vi "WSVCAP SHL Host LL RFFE Build and Parse Data.vi"(0 "Data Out":string, 1 "Data Out (Cycle Commands)":string[](array[string]), 2 "Post Command Delay":dbl[](array[numeric]) format="%#.0p s", 7 "Clock Rate (Hz) (Cycle Only)":dbl=50000.0, 9 "RFFE Data In [U8]":u8[][](array[numeric]) format="%02x", 12 "Simulate FPGA (Cycle Only)":bool, 13 "DUT Mask (All)":bool[](array[boolean])=[TRUE, TRUE, TRUE, TRUE, TRUE, TRUE, TRUE, TRUE, TRUE, TRUE, TRUE, TRUE, TRUE, TRUE, TRUE, TRUE, TRUE, TRUE, TRUE, TRUE, TRUE, TRUE, TRUE, TRUE, TRUE, TRUE, TRUE, TRUE, TRUE, TRUE, TRUE, TRUE, TRUE, TRUE, TRUE, TRUE, TRUE, TRUE, TRUE, TRUE, TRUE, TRUE, TRUE, TRUE, TRUE, TRUE, TRUE, TRUE, TRUE, TRUE, TRUE, TRUE, TRUE, TRUE, TRUE, TRUE, TRUE, TRUE, TRUE, TRUE, TRUE, TRUE, TRUE, TRUE]) -> (4 "RFFE Data Out [U8]":u8[][](array[numeric]) format="%02x", 6 "CMD Lengths (Bits)":u8[](array[numeric]), 8 "CMD Delays (Ticks)":u32[](array[numeric]), 10 "RFFE Data In":string[](array[string]))   [LabVIEW 2017]
panel:
  # "DUT 01"
  # "DUT 02"
  # "DUT 03"
  # "DUT 04"
  # "DUT 05"
  # "DUT 06"
  # "DUT 07"
  # "DUT 08"
  # "DUT 09"
  # "DUT 10"
  # "DUT 11"
  # "DUT 12"
  # "DUT 13"
  # "DUT 14"
  # "DUT 15"
  # "DUT 16"
  # "DUT 17"
  # "DUT 18"
  # "DUT 19"
  # "DUT 20"
  # "DUT 21"
  # "DUT 22"
  # "DUT 23"
  # "DUT 24"
  # "DUT 25"
  # "DUT 26"
  # "DUT 27"
  # "DUT 28"
  # "DUT 29"
  # "DUT 30"
  # "DUT 31"
  # "DUT 32"
  # "DUT 33"
  # "DUT 34"
  # "DUT 35"
  # "DUT 36"
  # "DUT 37"
  # "DUT 38"
  # "DUT 39"
  # "DUT 40"
  # "DUT 41"
  # "DUT 42"
  # "DUT 43"
  # "DUT 44"
  # "DUT 45"
  # "DUT 46"
  # "DUT 47"
  # "DUT 48"
  # "DUT 49"
  # "DUT 50"
  # "DUT 51"
  # "DUT 52"
  # "DUT 53"
  # "DUT 54"
  # "DUT 55"
  # "DUT 56"
  # "DUT 57"
  # "DUT 58"
  # "DUT 59"
  # "DUT 60"
  # "DUT 61"
  # "DUT 62"
  # "DUT 63"
  # "DUT 64"
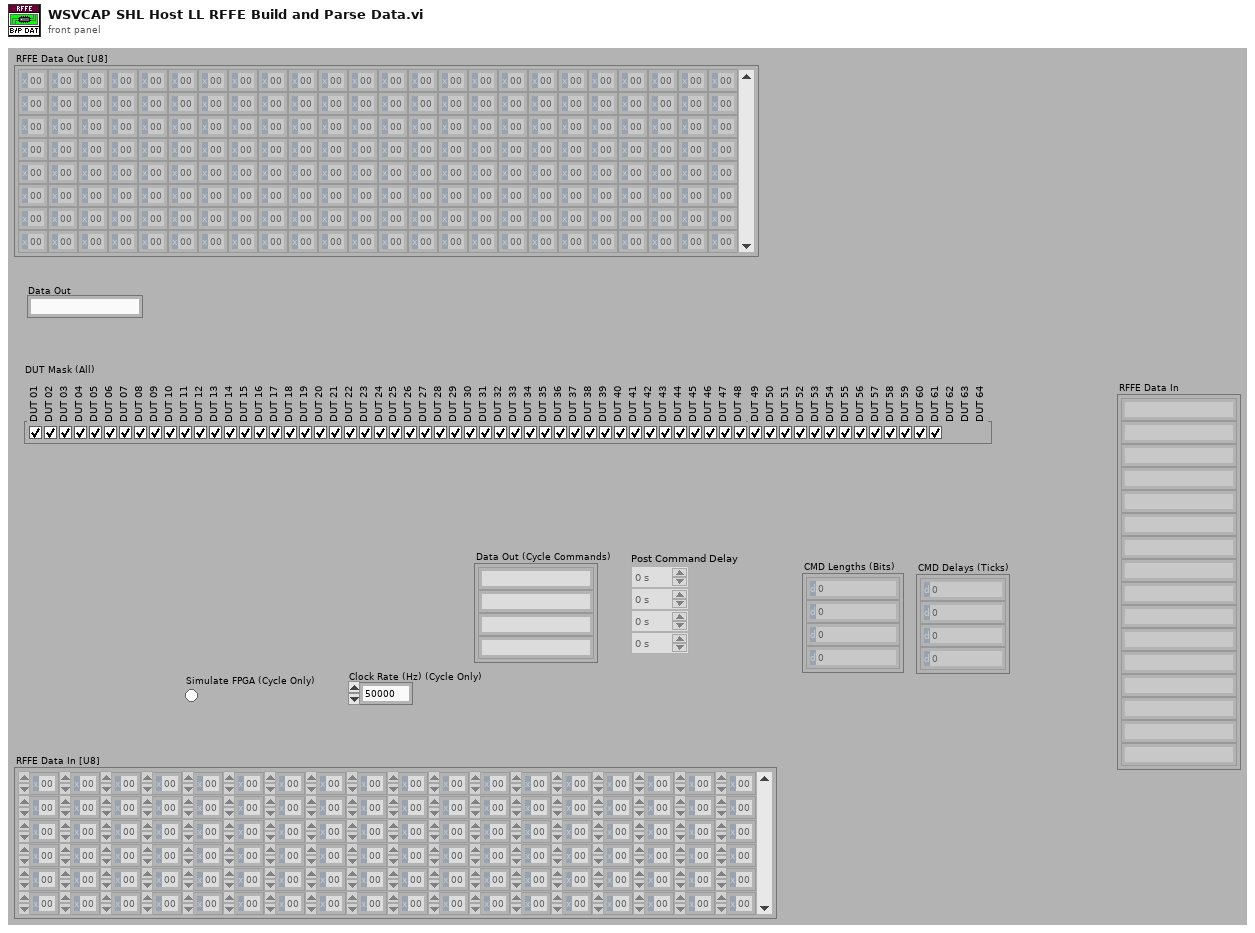
[diagram p1: front panel]
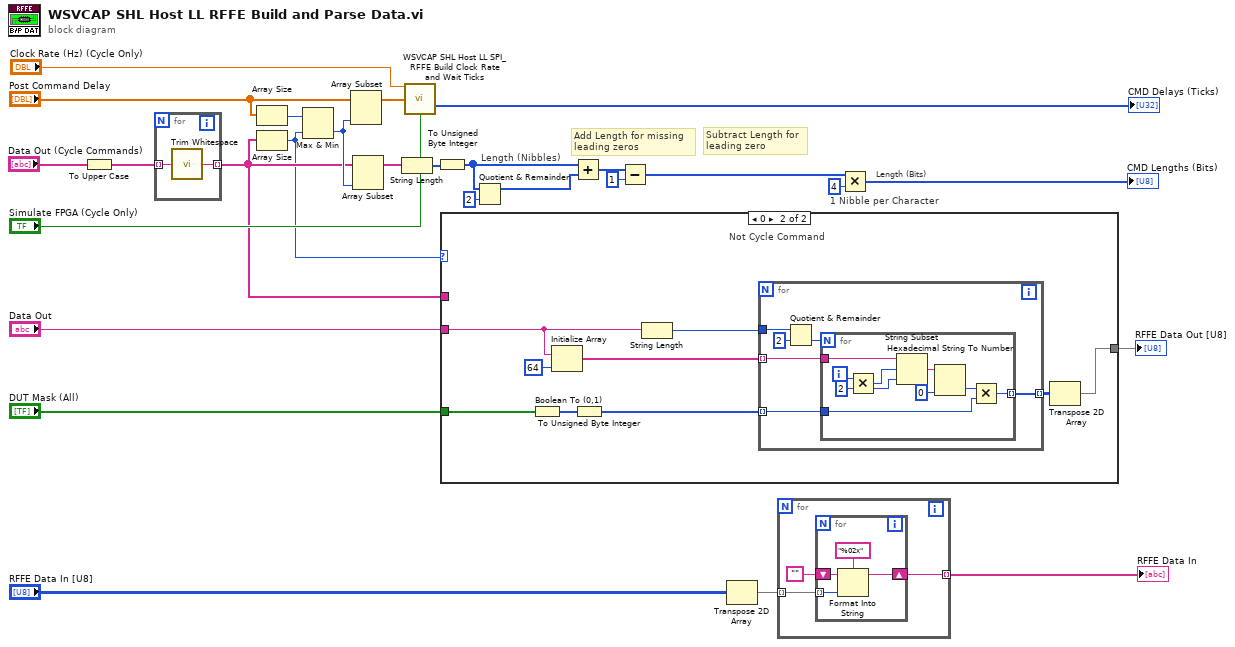
[diagram p0: block diagram]
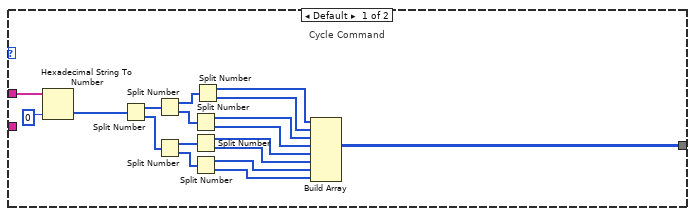
[diagram p2: hidden frame]
diagram:
  # "Subtract Length for\nleading zero"
  # "Add Length for missing\nleading zeros"
  # "Length (Bits)"
  # "Length (Nibbles)"
  # "1 Nibble per Character"
  n1 = To Upper Case(1:"Data Out (Cycle Commands)") -> (0:w2:string[])
  n2 = for {
    tunnel: w2 -> [w29] mode=indexing
    tunnel: [w28] -> w12 mode=indexing
    n3 = call <vilib>:"Trim Whitespace.vi"("string"=w29) -> ("trimmed string"=w28:string)  [unwired: 1 in]
  }
  n4 = Array Size(array="Post Command Delay") -> (size(s)=w21:i32)
  n5 = Array Size(array=w12) -> (size(s)=w11:i32)
  n6 = Max & Min(x=w21, y=w11) -> (min(x,y)=w18:i32)  [unwired: 1 out]
  n7 = Array Subset(array="Post Command Delay", length=w18) -> (w19:dbl[])  [unwired: 1 in]
  n8 = Array Subset(array=w12, length=w18) -> (w17:string[])  [unwired: 1 in]
  n9 = String Length(string=w17) -> (length=w23:i32[])
  n10 = call "WSVCAP SHL Host LL SPI_RFFE Build Clock Rate and Wait Ticks.vi"("Clock Rate (Hz)"="Clock Rate (Hz) (Cycle Only)", "CMD Delay (s)"=w19, "Simulate FPGA"="Simulate FPGA (Cycle Only)") -> ("CMD Delay (Ticks)"=→"CMD Delays (Ticks)":u32[])  [unwired: 9 in, 3 out]
  n11 = To Unsigned Byte Integer(number=w23) -> (unsigned 8bit integer=w8:u8[])
  n12 = case shown="0" w11 {
    tunnel: "DUT Mask (All)" -> [_ w56]
    tunnel: [w30 w51] -> w24
    tunnel: "Data Out" -> [_ w49]
    tunnel: w12 -> [w47 _]
    frame Default {
      # "Cycle Command"
      n13 = Hexadecimal String To Number(string=w47, default (0uL)=u64 0 ("Read Data")) -> (number=w40:u64[])  [unwired: 1 in, 1 out]
      n14 = Split Number(x=w40) -> (hi(x)=w45:u32[], lo(x)=w44:u32[])
      n15 = Split Number(x=w45) -> (hi(x)=w33:u16[], lo(x)=w43:u16[])
      n16 = Split Number(x=w44) -> (hi(x)=w42:u16[], lo(x)=w41:u16[])
      n17 = Split Number(x=w43) -> (hi(x)=w34:u8[], lo(x)=w39:u8[])
      n18 = Split Number(x=w42) -> (hi(x)=w38:u8[], lo(x)=w37:u8[])
      n19 = Split Number(x=w41) -> (hi(x)=w36:u8[], lo(x)=w35:u8[])
      n20 = Split Number(x=w33) -> (hi(x)=w31:u8[], lo(x)=w32:u8[])
      n21 = Build Array(w31, w32, w34, w39, w38, w37, w36, w35) -> (w30:u8[][])
    }
    frame 0 {
      # "Not Cycle Command"
      n22 = Boolean To (0,1)(Boolean=w56) -> (0, 1=w55:i16[])
      n23 = Initialize Array(w49, 64 ("dimension size")) -> (w50:string[])
      n24 = To Unsigned Byte Integer(number=w55) -> (unsigned 8bit integer=w54:u8[])
      n25 = String Length(string=w49) -> (length=w48:i32)
      n26 = for {
        tunnel: w54 -> [w60] mode=indexing
        tunnel: [w59] -> w53 mode=indexing
        tunnel: w50 -> [w58] mode=indexing
        tunnel: w48 -> [w57]
        n27 = Quotient & Remainder(x=w57, y=2) -> (floor(x/y)=w61:i32)  [unwired: 1 out]
        n28 = for {
          N: w61 -> [_]
          tunnel: w58 -> [w71]
          tunnel: [w64] -> w59 mode=indexing
          tunnel: w60 -> [w65]
          i -> [w70]
          w68 = 2 ("y")
          n29 = Multiply(x=w70, y=w68) -> (x*y=w69:i32)
          n30 = String Subset(string=w71, offset (0)=w69, length (rest)=w68) -> (substring=w67:string)
          n31 = Hexadecimal String To Number(string=w67, default (0uL)=u8 0 ("default (0 U32)")) -> (number=w63:u8)  [unwired: 1 in, 1 out]
          n32 = Multiply(x=w63, y=w65) -> (x*y=w64:u8)
        }
      }
      n33 = Transpose 2D Array(2D array=w53) -> (transposed array=w51:u8[][])
    }
  }
  "RFFE Data Out [U8]" <- w24
  n34 = Quotient & Remainder(x=w8, y=u8 2) -> (x-y*floor(x/y)=w7:u8[])  [unwired: 1 out]
  n35 = Add(x=w8, y=w7) -> (x+y=w5:u8[])
  n36 = Subtract(x=w5, y=u8 1 ("Read Data")) -> (x-y=w1:u8[])
  n37 = Transpose 2D Array(2D array="RFFE Data In [U8]") -> (transposed array=w26:u8[][])
  n38 = for {
    tunnel: w26 -> [w74] mode=indexing
    tunnel: [w72] -> w25 mode=indexing
    n39 = for {
      tunnel: w74 -> [w78] mode=indexing
      shift-right: [w76] -> w72
      shift-left: "" -> [w75]
      n40 = Format Into String(format string="%02x", initial string=w75, w78) -> (resulting string=w76:string)  [unwired: 1 in, 1 out]
    }
  }
  "RFFE Data In" <- w25
  n41 = Multiply(x=w1, y=u8 4 ("Read Data")) -> (x*y=→"CMD Lengths (Bits)":u8[])
